vi "read_params.vi"(8 "error in (no error)":errorcluster, 11 "GaussianProcessClassifier in":refnum<class "GaussianProcessClassifier.lvclass">) -> (0 "error out":errorcluster, 2 "params":T1={"n_restarts_optimizer"=0.0, "max_iter_predict"=0.0, "warm_start"=FALSE, "copy_X_train"=TRUE, "random_state"=0.0, "multi_class"="one_vs_rest", "n_jobs"=1.0}, 3 "GaussianProcessClassifier out":refnum<class "GaussianProcessClassifier.lvclass">)   [LabVIEW 2020, in "GaussianProcessClassifier.lvclass"]
uses:
  GaussianProcessClassifier.lvclass
  Controls/gaussian_process_classifier_params.ctl
  GaussianProcessClassifier.lvclass/GaussianProcessClassifier.ctl
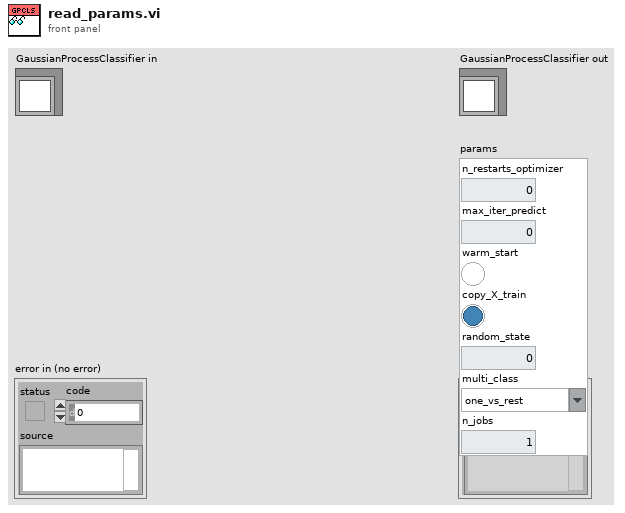
[diagram p1: front panel]
types:
  T1 = typedef "gaussian_process_classifier_params.ctl" = cluster{"n_restarts_optimizer":dbl, "max_iter_predict":dbl, "warm_start":bool, "copy_X_train":bool, "random_state":dbl, "multi_class":string, "n_jobs":dbl}
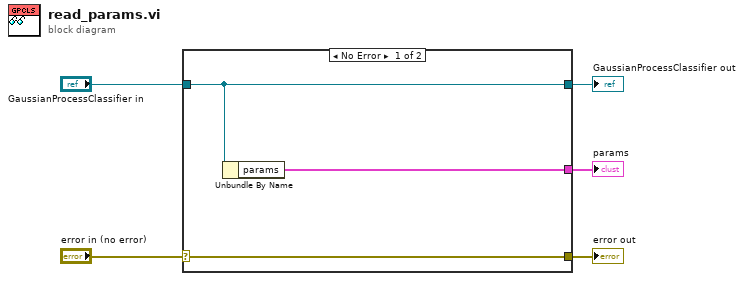
[diagram p0: block diagram]
diagram:
  n1 = case shown="No Error" "error in (no error)" {
    selector: "error in (no error)" -> [w8 w9]
    tunnel: [w8 w9] -> w4
    tunnel: [w7 w10] -> w2
    tunnel: "GaussianProcessClassifier in" -> [w7 w10]
    tunnel: [w6 _] -> w1
    frame No Error {
      n2 = Unbundle By Name(w7) -> ("params"=w6:T1)
    }
    frame Error {
    }
  }
  "error out" <- w4
  "GaussianProcessClassifier out" <- w2
  "params" <- w1
